vi "文件夹路径.vi"() -> (3 "appended path":path)   [LabVIEW 2018]
uses:
  <vilib>/Utility/sysdir.llb/System Directory Type.ctl
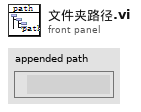
[diagram p1: front panel]
types:
  T1 = typedef "System Directory Type.ctl" = i32
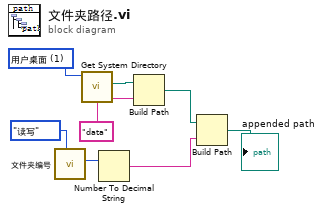
[diagram p0: block diagram]
diagram:
  w1 = T1 1 items=["用户目录"=0, "用户桌面"=1, "用户文档"=2, "用户应用程序数据"=3, "用户设置"=4, "用户临时目录"=5, "公共文档"=6, "公共应用程序数据"=7, "公共设置"=8, "公共缓存"=13, "系统核心库"=9, "系统安装库"=10, "应用程序文件"=11, "启动盘根目录"=12] ("system directory type")
  n1 = call "文件夹编号.vi"("模式"=enum16{"读", "写", "读写"}."读写") -> ("文件夹序号out"=w7:u32)  [unwired: 9 in, 1 out]
  n2 = call <vilib>:"Get System Directory.vi"("system directory type"=w1) -> ("system directory"=w2:path)  [unwired: 10 in]
  n3 = Number To Decimal String(number=w7) -> (decimal integer string=w8:string)  [unwired: 1 in]
  n4 = Build Path(base path=w2, name or relative path="data" ("名称或相对路径")) -> (appended path=w4:path)
  n5 = Build Path(base path=w4, name or relative path=w8) -> (appended path=→"appended path":path)
